vi "single_tone_analysis.vi"(11 "channels":tag="Dev2/ai4:7") -> (1 "Phases":dbl[](array[numeric]), 2 "Amps":dbl[](array[numeric]), 3 "Freqs":dbl[](array[numeric]))   [LabVIEW 2014]
uses:
  <vilib>/DAQmx/create/channels.llb/DAQmx Create Channel (AI-Voltage-Basic).vi
  <vilib>/DAQmx/configure/timing.llb/DAQmx Timing (Sample Clock).vi
  <vilib>/DAQmx/read.llb/DAQmx Read (Analog 1D Wfm NChan NSamp).vi
  <vilib>/measure/matone.llb/Extract Single Tone Information N Chan.vi
  <vilib>/measure/NI_MAPro.lvlib
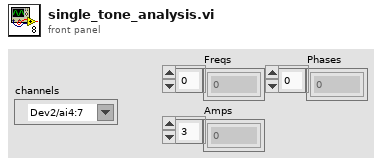
[diagram p1: front panel]
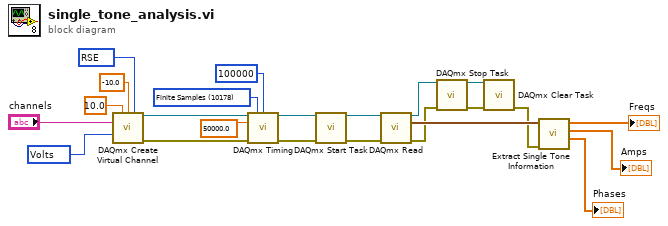
[diagram p0: block diagram]
diagram:
  w17 = 10178 items=["Finite Samples"=10178, "Continuous Samples"=10123, "Hardware Timed Single Point"=12522] ("sample mode")
  w19 = 10083 items=["default"=-1, "RSE"=10083, "NRSE"=10078, "Differential"=10106, "Pseudodifferential"=12529] ("input terminal configuration")
  w21 = 10348 items=["Volts"=10348, "From Custom Scale"=10065] ("units")
  n1 = call-poly <vilib>:"DAQmx Create Virtual Channel.vi"("maximum value"=10.0, "minimum value"=-10.0, "input terminal configuration"=w19, "physical channels"="channels", "units"=w21) -> ("task out"=w14:refnum<k21>, "error out"=w6:errorcluster)  [unwired: 9 in]
  n2 = call-poly <vilib>:"DAQmx Timing.vi"("task/channels in"=w14, "sample mode"=w17, "samples per channel"=100000, "rate"=50000.0, "error in"=w6) -> ("task out"=w13:refnum<k21>, "error out"=w5:errorcluster)  [unwired: 9 in]
  n3 = call <vilib>:"DAQmx Start Task.vi"("task/channels in"=w13, "error in"=w5) -> ("task out"=w20:refnum<k21>, "error out"=w4:errorcluster)  [unwired: 12 in]
  n4 = call-poly <vilib>:"DAQmx Read.vi"("task/channels in"=w20, "error in"=w4) -> ("task out"=w3:refnum<k21>, "data"=w12:waveform(dbl)[], "error out"=w2:errorcluster)  [unwired: 11 in]
  n5 = call <vilib>:"DAQmx Stop Task.vi"("task/channels in"=w3, "error in"=w2) -> ("task out"=w7:refnum<k21>, "error out"=w8:errorcluster)  [unwired: 12 in]
  n6 = call <vilib>:"DAQmx Clear Task.vi"("task in"=w7, "error in"=w8) -> ("error out"=w1:errorcluster)  [unwired: 13 in]
  n7 = call-poly <vilib>:"Extract Single Tone Information.vi"("error in (no error)"=w1, "time signals in"=w12) -> ("detected phases (deg)"=→"Phases":dbl[], "detected amplitudes"=→"Amps":dbl[], "detected frequencies"=→"Freqs":dbl[])  [unwired: 4 in, 3 out]
